vi "Tick Period to RPM.vi"(10 "Tick Period":u32) -> (2 "nWheel":fxp<+/-,32,16>)   [LabVIEW 2014]
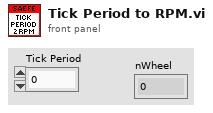
[diagram p1: front panel]
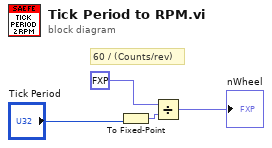
[diagram p0: block diagram]
diagram:
  # "60 / (Counts/rev)"
  n1 = To Fixed-Point(number="Tick Period") -> (fixed-point=w2:fxp<+,32,16>)  [unwired: 1 in]
  n2 = Divide(x=fxp<+,1,3> 4.0, y=w2) -> (x/y=→"nWheel":fxp<+/-,32,16>)
